vi "test_example_4.vi"() -> ()   [LabVIEW 2014]
uses:
  build/example_4.dll
panel:
  out "return type":u64
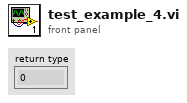
[diagram p1: front panel]
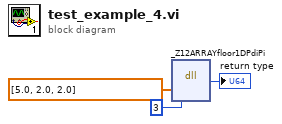
[diagram p0: block diagram]
diagram:
  n1 = dll-call lib="C:/Users/Simon Gurfunkel/Documents/LabVIEW_projects/LabVIEW-Transcript-DLL-Library/examples/4/build/example_4.dll" fn="_Z12ARRAYfloor1DPdiPi"("arg1"=dbl[] [5.0, 2.0, 2.0], "arg2"=3) -> ("return type"=→"return type":u64)  [unwired: 5 in, 2 out]
